vi "usbpt104+usbTC-arduino control PWM (RTD-TC PID).vi"() -> ()   [LabVIEW 2015]
uses:
  <vilib>/MakerHub/LINX/Public/Peripherals/Digital/Digital Write 1 Chan.vi
  <vilib>/MakerHub/LINX/Public/Peripherals/Digital/Digital Write N Chans.vi
  <vilib>/MakerHub/LINX/Private/Local IO/LinxDigitalWrite.vi
  <vilib>/MakerHub/LINX/Public/Utilities/Check Channel.vi
  Instance           1 16Saved   USBPT104 .vi
  <vilib>/MakerHub/LINX/Private/Utilties/Generate Error.vi
  <vilib>/MakerHub/LINX/LMH-LINX.lvlib
  UsbPT104.dll
  usbtc08.dll
panel:
  in  "RTD":bool
  out "Temperature":sgl
  out "RTD 4":dbl(slide) max=10000.0 scale=-200.0..800.0
  out "RTD 3":dbl(slide) max=10000.0 scale=-200.0..800.0
  out "RTD 2":dbl(slide) max=10000.0 scale=-200.0..800.0
  in  "PT104 Connection":bool=TRUE
  in  "IP Address":string
  out "Low Pulse Duration (ms)":dbl
  in  "Relay I/O Pin":u8
  in  "Update settings":bool
  in  "Stop":bool
  in  "PID":T1={"proportional gain (Kc)"=5.0, "integral time (Ti, min)"=0.0, "derivative time (Td, min)"=0.0}
  out "Data Saving...":bool caption="Saving Data"
  in  "Enable Save?":bool=TRUE caption="Enable"
  out "CH 8":sgl
  out "CH 7":sgl
  out "CH 6":sgl
  out "CH 5":sgl
  out "CH 4":sgl
  out "CH 3":sgl
  out "CH 2":sgl
  out "CH 1":sgl
  out "CH 0":sgl
  in  "Mains Frequency":i16(ring) items=["50 Hz", "60 Hz"]
  out "Handle":i16
  in  "?":bool
  in  "Units":enum16{"C°", "F°", "K°", "R°"}(ring)
  in  "Ch # 8":bool
  in  "Type # 8":i16(ring)=107 items=["B"=98, "E"=101, "J"=106, "K"=107, "N"=110, "R"=114, "S"=115, "T"=116, "Voltage"=120]
  in  "Ch # 7":bool
  in  "Type # 7":i16(ring)=107 items=["B"=98, "E"=101, "J"=106, "K"=107, "N"=110, "R"=114, "S"=115, "T"=116, "Voltage"=120]
  in  "Ch # 6":bool
  in  "Type # 6":i16(ring)=107 items=["B"=98, "E"=101, "J"=106, "K"=107, "N"=110, "R"=114, "S"=115, "T"=116, "Voltage"=120]
  in  "Ch # 5":bool
  in  "Type # 5":i16(ring)=107 items=["B"=98, "E"=101, "J"=106, "K"=107, "N"=110, "R"=114, "S"=115, "T"=116, "Voltage"=120]
  in  "Ch # 4":bool
  in  "Type # 4":i16(ring)=107 items=["B"=98, "E"=101, "J"=106, "K"=107, "N"=110, "R"=114, "S"=115, "T"=116, "Voltage"=120]
  in  "Ch # 3":bool
  in  "Type # 3":i16(ring)=107 items=["B"=98, "E"=101, "J"=106, "K"=107, "N"=110, "R"=114, "S"=115, "T"=116, "Voltage"=120]
  in  "Ch# 2":bool=TRUE
  in  "Type # 2":i16(ring)=107 items=["B"=98, "E"=101, "J"=106, "K"=107, "N"=110, "R"=114, "S"=115, "T"=116, "Voltage"=120]
  in  "Ch# 1":bool=TRUE
  in  "Type # 1":i16(ring)=107 items=["B"=98, "E"=101, "J"=106, "K"=107, "N"=110, "R"=114, "S"=115, "T"=116, "Voltage"=120]
  in  "Arduino Comms Port":refnum<visa-resource-name>
  out "Pulse Duration (ms)":dbl
  in  "Duty Cycle Period (ms)":u32=1000
  out "Duty Cycle (%)":dbl format="%.2f"
  out "PWM":dynamicdata(graph) caption="Square"
  in  "PID Temp Setpoint":u16=13
  out "?":dynamicdata(graph)
  in  "CH4 Measurement Type":i32(ring) items=["OFF", "PT100", "PT1000", "Resistance to 375 Ohms", "Resistance to 10 kOhms", "Differential to 115 mV", "Differential to 2500 mV", "Single-ended to 115 mV", "Single-ended to 2500 mV"]
  in  "CH4 Number of Wires":i16(ring)=4 items=["2"=2, "3"=3, "4"=4]
  in  "CH3 Measurement Type":i32(ring) items=["OFF", "PT100", "PT1000", "Resistance to 375 Ohms", "Resistance to 10 kOhms", "Differential to 115 mV", "Differential to 2500 mV", "Single-ended to 115 mV", "Single-ended to 2500 mV"]
  in  "CH3 Number of Wires":i16(ring)=4 items=["2"=2, "3"=3, "4"=4]
  in  "CH2 Measurement Type":i32(ring) items=["OFF", "PT100", "PT1000", "Resistance to 375 Ohms", "Resistance to 10 kOhms", "Differential to 115 mV", "Differential to 2500 mV", "Single-ended to 115 mV", "Single-ended to 2500 mV"]
  in  "CH2 Number of Wires":i16(ring)=4 items=["2"=2, "3"=3, "4"=4]
  in  "CH1 Number of Wires":i16(ring)=2 items=["2"=2, "3"=3, "4"=4]
  in  "CH1 Measurement Type":i32(ring)=1 items=["OFF", "PT100", "PT1000", "Resistance to 375 Ohms", "Resistance to 10 kOhms", "Differential to 115 mV", "Differential to 2500 mV", "Single-ended to 115 mV", "Single-ended to 2500 mV"]
  out "RTD 1":dbl(slide) max=10000.0 scale=-200.0..800.0
  # "RTD Channel 1 (PID Driven)"
  # "RTD Channel 2"
  # "RTD Channel 3"
  # "RTD Channel 4"
  # "TC"
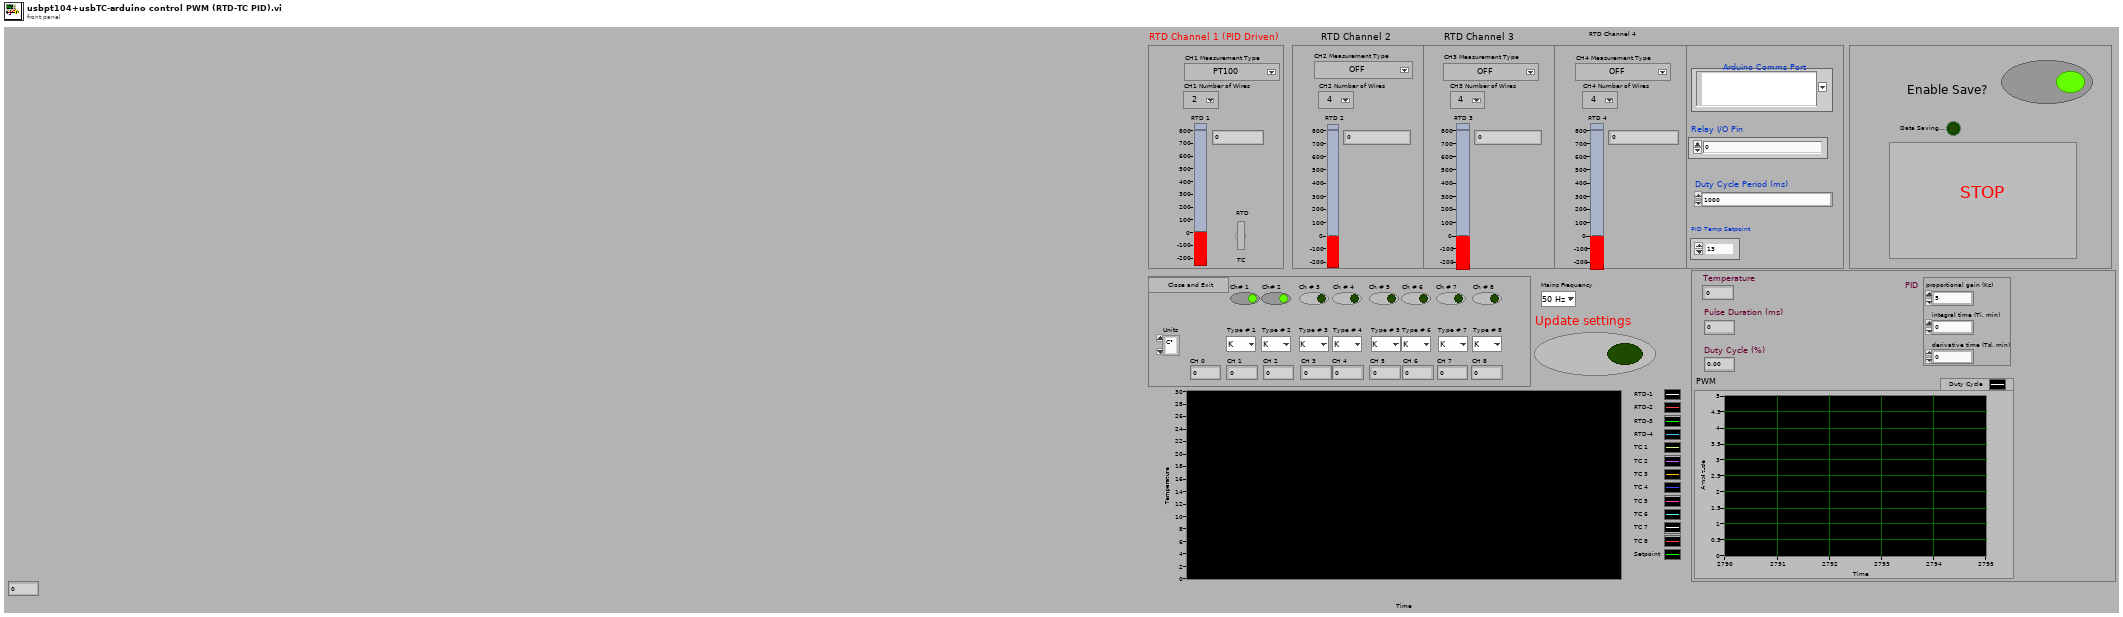
[diagram p1: front panel]
types:
  T1 = cluster{"proportional gain (Kc)":dbl, "integral time (Ti, min)":dbl, "derivative time (Td, min)":dbl}
  T2 = typedef "LMH-LINX.lvlib/LINX Ref.ctl" = cluster{"IO":T3, "Interface":T4, "LINX Device Config":T5}
  T3 = typedef "LMH-LINX.lvlib/Platform.ctl" = enum16{"Remote", "Local"}
  T4 = typedef "LMH-LINX.lvlib/Interface.ctl" = enum16{"Serial", "TCP"}
  T5 = typedef "LMH-LINX.lvlib/Device.lvlib/LINX Device Config.ctl" = cluster{"Interface":T4, "COM Port":refnum<visa-resource-name>, "TCP Configuration":T6, "Device Family":u8, "Device ID":u8, "Device Name":string, "TCP Ref":refnum<k5>, "Channels":T7}
  T6 = typedef "LMH-LINX.lvlib/Device.lvlib/TCP Config.ctl" = cluster{"IP Address":string, "Port":u16}
  T7 = typedef "LMH-LINX.lvlib/Channels.ctl" = cluster{"DI":u8[], "DO":u8[], "AI":u8[], "AO":u8[], "PWM":u8[], "QE":u8[], "UART":u8[], "I2C 2":u8[], "SPI":u8[], "CAN":u8[], "Servo":u8[], "AI Ref (V)":dbl, "AI Resolution (Bits)":u8, "AO Ref (V)":dbl, "AO Resolution (Bits)":u8}
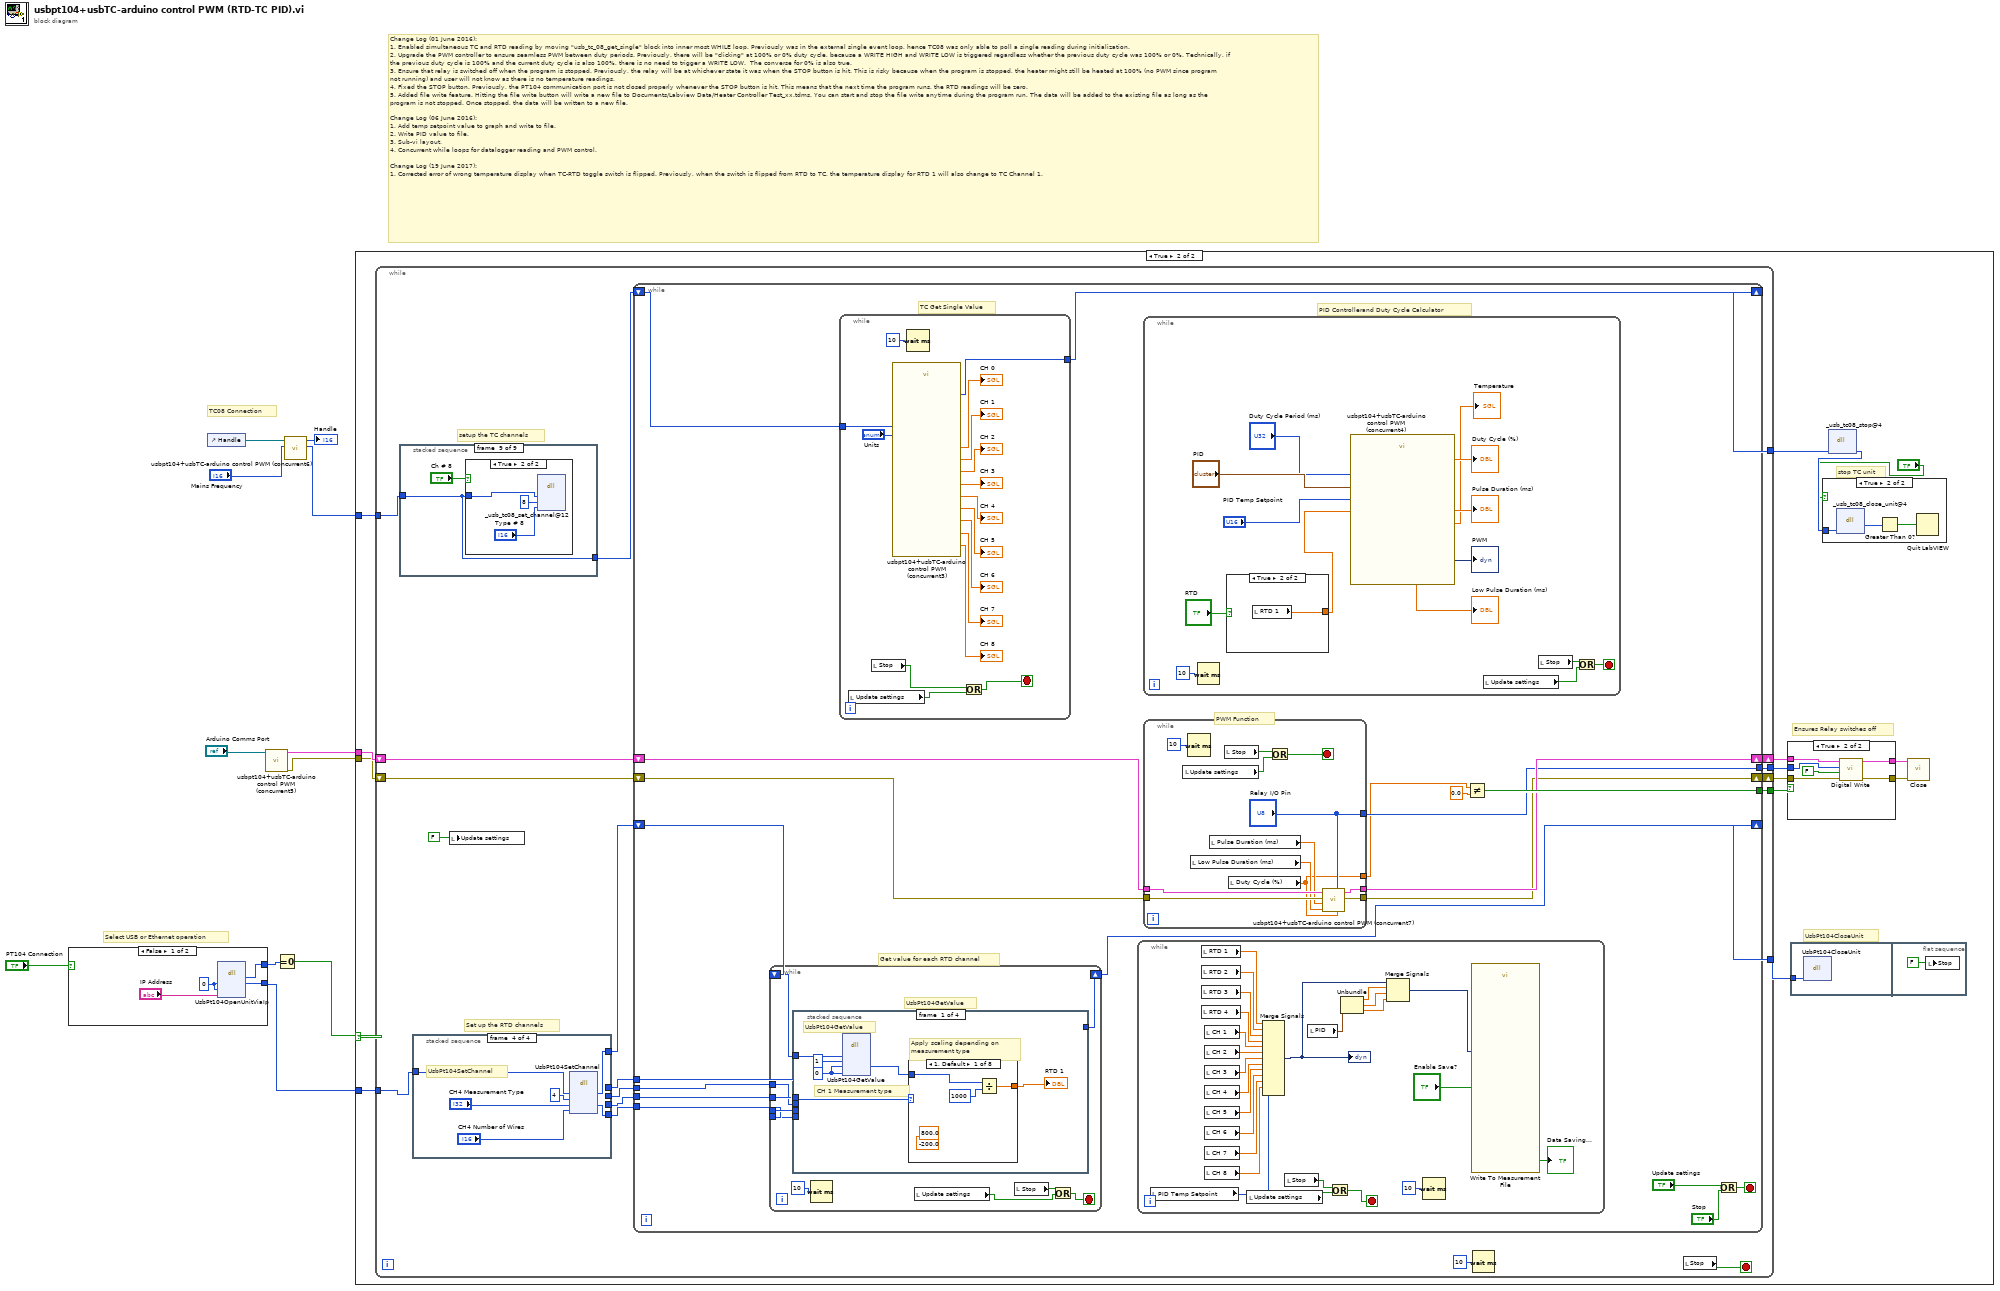
[diagram p0: block diagram]
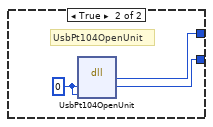
[diagram p2: hidden frame]
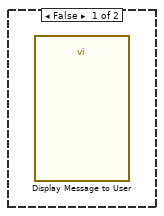
[diagram p3: hidden frame]
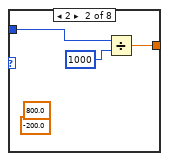
[diagram p4: hidden frame]
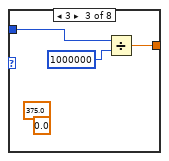
[diagram p5: hidden frame]
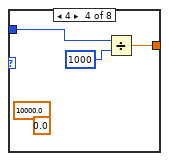
[diagram p6: hidden frame]
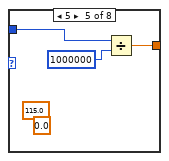
[diagram p7: hidden frame]
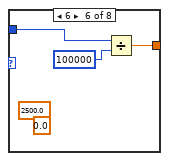
[diagram p8: hidden frame]
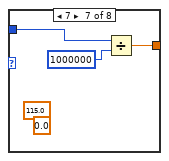
[diagram p9: hidden frame]
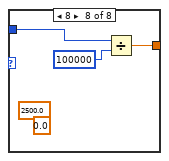
[diagram p10: hidden frame]
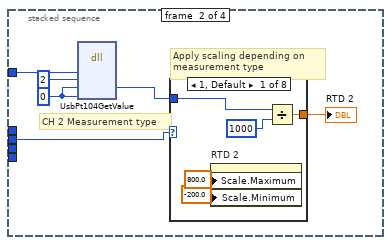
[diagram p11: hidden frame]
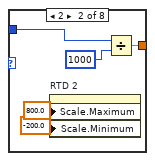
[diagram p12: hidden frame]
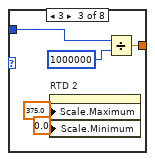
[diagram p13: hidden frame]
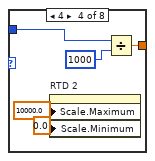
[diagram p14: hidden frame]
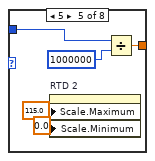
[diagram p15: hidden frame]
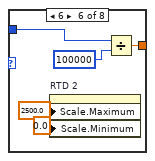
[diagram p16: hidden frame]
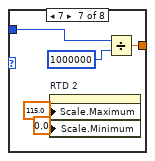
[diagram p17: hidden frame]
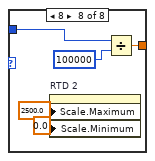
[diagram p18: hidden frame]
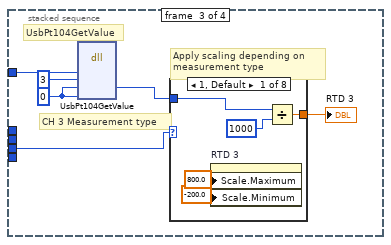
[diagram p19: hidden frame]
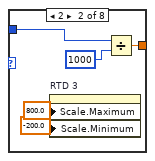
[diagram p20: hidden frame]
diagram:
  # "Select USB or Ethernet operation"
  # "TC08 Connection"
  # "Change Log (01 June 2016):\n1. Enabled simultaneous TC and RTD reading by moving \"usb_tc_08_get_single\" block into inner most WHILE loop. Previously was in the external single event loop, hence TC08 was only able to poll a single reading during initialization.\n2. Upgrade the PWM controller to ensure seamless PWM between duty periods. Previously, there will be \"clicking\" at 100% or 0% duty cycle, because a WRITE HIGH and WRITE LOW is triggered regardless whether the previous duty cycle was 100% or 0%. Technically, if the previous duty cycle is 100% and the current duty cycle is also 100%, there is no need to trigger a WRITE LOW.  The converse for 0% is also true. \n3. Ensure that relay is switched off when the program is stopped. Previously, the relay will be at whichever state it was when the STOP button is hit. This is risky because when the program is stopped, the heater might still be heated at 100% (no PWM since program not running) and user will not know as there is no temperature readings.\n4. Fixed the STOP button. Previously, the PT104 communication port is not closed properly whenever the STOP button is hit. This means that the next time the program runs, the RTD readings will be zero.\n5. Added file write feature. Hitting the file write button will write a new file to Documents/Labview Data/Heater Controller Test_xx.tdms. You can start and stop the file write anytime during the program run. The data will be added to the existing file as long as the program is not stopped. Once stopped, the data will be written to a new file. \n\nChange Log (06 June 2016):\n1. Add temp setpoint value to graph and write to file.\n2. Write PID value to file.\n3. Sub-vi layout.\n4. Concurrent while loops for datalogger reading and PWM control.\n\nChange Log (19 June 2017):\n1. Corrected error of wrong temperature display when TC-RTD toggle switch is flipped. Previously, when the switch is flipped from RTD to TC, the temperature display for RTD 1 will also change to TC Channel 1."
  n1 = case shown="False" "PT104 Connection" {
    tunnel: [w13 w18] -> w3
    tunnel: [w12 w17] -> w2
    frame False {
      w15 = i16 0 ("handle")
      n2 = dll-call lib="UsbPT104.dll" fn="UsbPt104OpenUnitViaIp"("handle"=w15, "serial"=w15, "IpAddress"="IP Address") -> ("Status"=w13:i32, "handle"=w12:i16)  [unwired: 5 in, 2 out]
    }
    frame True {
      w16 = i16 0 ("handle")
      # "UsbPt104OpenUnit"
      n3 = dll-call lib="UsbPT104.dll" fn="UsbPt104OpenUnit"("handle"=w16, "serial"=w16) -> ("Status"=w18:i32, "handle"=w17:i16)  [unwired: 4 in, 2 out]
    }
  }
  n4 = control-ref of="Handle"() -> (w9:refnum<vi>)
  n5 = call "usbpt104+usbTC-arduino control PWM (concurrent5).vi"("Arduino Comms Port"="Arduino Comms Port") -> ("error out"=w5:errorcluster, "LINX Resource"=w6:T2)  [unwired: 8 in]
  n6 = Equal To 0?(x=w3) -> (x = 0?=w1:bool)
  n7 = call "usbpt104+usbTC-arduino control PWM (concurrent6).vi"("Mains Frequency"="Mains Frequency", "Digital in"=w9) -> ("Handle 2"=w7:i16, "Handle"=→"Handle":i16)  [unwired: 8 in]
  n8 = case shown="True" w1 {
    tunnel: w7 -> [_ w27]
    tunnel: w2 -> [_ w19]
    tunnel: w6 -> [_ w24]
    tunnel: w5 -> [_ w22]
    frame False {
      n9 = call "Display Message to User"() -> ()  [unwired: 10 in, 2 out]
    }
    frame True {
      # "Ensures Relay switches off"
      # "UsbPt104CloseUnit"
      # "stop TC unit"
      n10 = while {
        tunnel: [w51] -> w28
        tunnel: w27 -> [w45]
        tunnel: [w43] -> w26
        tunnel: [w42] -> w25
        tunnel: [w37] -> w20
        tunnel: w19 -> [w36]
        shift-right: [w40] -> w23
        shift-left: w24 -> [w41]
        shift-right: [w38] -> w21
        shift-left: w22 -> [w39]
        stop <- w35 stop-if-true
        # "Set up the RTD channels"
        # "setup the TC channels"
        n11 = stacked-sequence {
          tunnel: [_ _ _ _ _ _ _ _ w399] -> w44
          tunnel: w45 -> [w340 w343 w351 w359 w367 w375 w383 w391 w399]
          frame #0 {
            n12 = dll-call lib="usbtc08.dll" fn="_usb_tc08_set_channel@12"("handle"=w340, "channel"=i16 0, "tc_type"=i8 0) -> ()  [unwired: 7 in, 2 out]
          }
          frame #1 {
            n13 = case shown="True" "Ch# 1" {
              tunnel: w343 -> [w346 w348]
              frame False {
                n14 = dll-call lib="usbtc08.dll" fn="_usb_tc08_set_channel@12"("handle"=w346, "channel"=i16 1, "tc_type"=32) -> ()  [unwired: 7 in, 2 out]
              }
              frame True {
                n15 = dll-call lib="usbtc08.dll" fn="_usb_tc08_set_channel@12"("handle"=w348, "channel"=i16 1, "tc_type"="Type # 1") -> ()  [unwired: 7 in, 2 out]
              }
            }
          }
          frame #2 {
            n16 = case shown="False" "Ch# 2" {
              tunnel: w351 -> [w353 w357]
              frame False {
                n17 = dll-call lib="usbtc08.dll" fn="_usb_tc08_set_channel@12"("handle"=w353, "channel"=i16 2, "tc_type"=32) -> ()  [unwired: 7 in, 2 out]
              }
              frame True {
                n18 = dll-call lib="usbtc08.dll" fn="_usb_tc08_set_channel@12"("handle"=w357, "channel"=i16 2, "tc_type"="Type # 2") -> ()  [unwired: 7 in, 2 out]
              }
            }
          }
          frame #3 {
            n19 = case shown="True" "Ch # 3" {
              tunnel: w359 -> [w361 w365]
              frame False {
                n20 = dll-call lib="usbtc08.dll" fn="_usb_tc08_set_channel@12"("handle"=w361, "channel"=i16 3, "tc_type"=32) -> ()  [unwired: 7 in, 2 out]
              }
              frame True {
                n21 = dll-call lib="usbtc08.dll" fn="_usb_tc08_set_channel@12"("handle"=w365, "channel"=i16 3, "tc_type"="Type # 3") -> ()  [unwired: 7 in, 2 out]
              }
            }
          }
          frame #4 {
            n22 = case shown="False" "Ch # 4" {
              tunnel: w367 -> [w369 w373]
              frame False {
                n23 = dll-call lib="usbtc08.dll" fn="_usb_tc08_set_channel@12"("handle"=w369, "channel"=i16 4, "tc_type"=32) -> ()  [unwired: 7 in, 2 out]
              }
              frame True {
                n24 = dll-call lib="usbtc08.dll" fn="_usb_tc08_set_channel@12"("handle"=w373, "channel"=i16 4, "tc_type"="Type # 4") -> ()  [unwired: 7 in, 2 out]
              }
            }
          }
          frame #5 {
            n25 = case shown="False" "Ch # 5" {
              tunnel: w375 -> [w377 w380]
              frame False {
                n26 = dll-call lib="usbtc08.dll" fn="_usb_tc08_set_channel@12"("handle"=w377, "channel"=i16 5, "tc_type"=32) -> ()  [unwired: 7 in, 2 out]
              }
              frame True {
                n27 = dll-call lib="usbtc08.dll" fn="_usb_tc08_set_channel@12"("handle"=w380, "channel"=i16 5, "tc_type"="Type # 5") -> ()  [unwired: 7 in, 2 out]
              }
            }
          }
          frame #6 {
            n28 = case shown="False" "Ch # 6" {
              tunnel: w383 -> [w385 w389]
              frame False {
                n29 = dll-call lib="usbtc08.dll" fn="_usb_tc08_set_channel@12"("handle"=w385, "channel"=i16 6, "tc_type"=32) -> ()  [unwired: 7 in, 2 out]
              }
              frame True {
                n30 = dll-call lib="usbtc08.dll" fn="_usb_tc08_set_channel@12"("handle"=w389, "channel"=i16 6, "tc_type"="Type # 6") -> ()  [unwired: 7 in, 2 out]
              }
            }
          }
          frame #7 {
            n31 = case shown="False" "Ch # 7" {
              tunnel: w391 -> [w393 w397]
              frame False {
                n32 = dll-call lib="usbtc08.dll" fn="_usb_tc08_set_channel@12"("handle"=w393, "channel"=i16 7, "tc_type"=32) -> ()  [unwired: 7 in, 2 out]
              }
              frame True {
                n33 = dll-call lib="usbtc08.dll" fn="_usb_tc08_set_channel@12"("handle"=w397, "channel"=i16 7, "tc_type"="Type # 7") -> ()  [unwired: 7 in, 2 out]
              }
            }
          }
          frame #8 {
            n34 = case shown="True" "Ch # 8" {
              tunnel: w399 -> [w401 w405]
              frame False {
                n35 = dll-call lib="usbtc08.dll" fn="_usb_tc08_set_channel@12"("handle"=w401, "channel"=i16 8, "tc_type"=32) -> ()  [unwired: 7 in, 2 out]
              }
              frame True {
                n36 = dll-call lib="usbtc08.dll" fn="_usb_tc08_set_channel@12"("handle"=w405, "channel"=i16 8, "tc_type"="Type # 8") -> ()  [unwired: 7 in, 2 out]
              }
            }
          }
        }
        n37 = stacked-sequence {
          tunnel: w36 -> [w323 w328 w333 w339]
          tunnel: [_ _ _ w335] -> w49
          tunnel: [w319 _ _ _] -> w50
          tunnel: [_ w324 _ _] -> w47
          tunnel: [_ _ w329 _] -> w46
          tunnel: [_ _ _ w334] -> w48
          frame #0 {
            # "UsbPt104SetChannel"
            n38 = dll-call lib="UsbPT104.dll" fn="UsbPt104SetChannel"("handle"=w323, "channel"=1, "type"="CH1 Measurement Type", "noOfWires"="CH1 Number of Wires") -> ("type"=w319:i32)  [unwired: 7 in, 2 out]
          }
          frame #1 {
            n39 = dll-call lib="UsbPT104.dll" fn="UsbPt104SetChannel"("handle"=w328, "channel"=2, "type"="CH2 Measurement Type", "noOfWires"="CH2 Number of Wires") -> ("type"=w324:i32)  [unwired: 7 in, 2 out]
          }
          frame #2 {
            # "UsbPt104SetChannel"
            n40 = dll-call lib="UsbPT104.dll" fn="UsbPt104SetChannel"("handle"=w333, "channel"=3, "type"="CH3 Measurement Type", "noOfWires"="CH3 Number of Wires") -> ("type"=w329:i32)  [unwired: 7 in, 2 out]
          }
          frame #3 {
            # "UsbPt104SetChannel"
            n41 = dll-call lib="UsbPT104.dll" fn="UsbPt104SetChannel"("handle"=w339, "channel"=4, "type"="CH4 Measurement Type", "noOfWires"="CH4 Number of Wires") -> ("handle"=w335:i16, "type"=w334:i32)  [unwired: 6 in, 2 out]
          }
        }
        n42 = local write "Update settings"(FALSE ("Update settings")) -> ()
        n43 = while {
          tunnel: [w69] -> w51
          tunnel: w50 -> [w59]
          tunnel: w48 -> [w55]
          tunnel: w47 -> [w57]
          tunnel: w46 -> [w56]
          tunnel: [w62] -> w37
          shift-right: [w52] -> w42
          shift-left: w49 -> [w58]
          shift-right: [w67] -> w43
          shift-left: w44 -> [w68]
          shift-right: [w65] -> w40
          shift-left: w41 -> [w66]
          shift-right: [w63] -> w38
          shift-left: w39 -> [w64]
          stop <- w60 stop-if-true
          # "PID Controllerand Duty Cycle Calculator"
          # "PWM Function"
          # "TC Get Single Value"
          # "Get value for each RTD channel"
          n44 = while {
            tunnel: w59 -> [w80]
            tunnel: w57 -> [w78]
            tunnel: w56 -> [w77]
            tunnel: w55 -> [w76]
            shift-right: [w75] -> w52
            shift-left: w58 -> [w79]
            stop <- w72 stop-if-true
            # "UsbPt104GetValue"
            n45 = stacked-sequence {
              tunnel: w79 -> [w86 w116 w162 w209]
              tunnel: [_ _ _ w206] -> w75
              tunnel: w80 -> [w82 _ _ _]
              tunnel: w78 -> [_ w111 _ _]
              tunnel: w77 -> [_ _ w157 _]
              tunnel: w76 -> [_ _ _ w203]
              frame #0 {
                w84 = 0 ("value")
                # "CH 1 Measurement type"
                # "Apply scaling depending on \nmeasurement type"
                # "UsbPt104GetValue"
                n46 = dll-call lib="UsbPT104.dll" fn="UsbPt104GetValue"("handle"=w86, "channel"=1, "value"=w84, "filtered"=w84) -> ("value"=w83:i32)  [unwired: 7 in, 2 out]
                n47 = case shown="1, Default" w82 {
                  tunnel: w83 -> [w88 w91 w94 w97 w100 w103 w106 w109]
                  tunnel: [w87 w90 w93 w96 w99 w102 w105 w108] -> w81
                  frame 1, Default {
                    (unwired) -200.0 ("Scale.Range:Minimum")
                    (unwired) 800.0 ("Data Range:Maximum")
                    n48 = Divide(x=w88, y=1000) -> (x/y=w87:dbl)
                  }
                  frame 2 {
                    (unwired) -200.0 ("Scale.Range:Minimum")
                    (unwired) 800.0 ("Data Range:Maximum")
                    n49 = Divide(x=w91, y=1000) -> (x/y=w90:dbl)
                  }
                  frame 3 {
                    (unwired) 0.0 ("Scale.Range:Minimum")
                    (unwired) 375.0 ("Data Range:Maximum")
                    n50 = Divide(x=w94, y=1000000) -> (x/y=w93:dbl)
                  }
                  frame 4 {
                    (unwired) 0.0 ("Scale.Range:Minimum")
                    (unwired) 10000.0 ("Data Range:Maximum")
                    n51 = Divide(x=w97, y=1000) -> (x/y=w96:dbl)
                  }
                  frame 5 {
                    (unwired) 0.0 ("Scale.Range:Minimum")
                    (unwired) 115.0 ("Data Range:Maximum")
                    n52 = Divide(x=w100, y=1000000) -> (x/y=w99:dbl)
                  }
                  frame 6 {
                    (unwired) 0.0 ("Scale.Range:Minimum")
                    (unwired) 2500.0 ("Data Range:Maximum")
                    n53 = Divide(x=w103, y=100000) -> (x/y=w102:dbl)
                  }
                  frame 7 {
                    (unwired) 0.0 ("Scale.Range:Minimum")
                    (unwired) 115.0 ("Data Range:Maximum")
                    n54 = Divide(x=w106, y=1000000) -> (x/y=w105:dbl)
                  }
                  frame 8 {
                    (unwired) 0.0 ("Scale.Range:Minimum")
                    (unwired) 2500.0 ("Data Range:Maximum")
                    n55 = Divide(x=w109, y=100000) -> (x/y=w108:dbl)
                  }
                }
                "RTD 1" <- w81
              }
              frame #1 {
                w114 = 0 ("value")
                # "CH 2 Measurement type"
                # "Apply scaling depending on \nmeasurement type"
                n56 = dll-call lib="UsbPT104.dll" fn="UsbPt104GetValue"("handle"=w116, "channel"=2, "value"=w114, "filtered"=w114) -> ("value"=w113:i32)  [unwired: 7 in, 2 out]
                n57 = case shown="1, Default" w111 {
                  tunnel: w113 -> [w120 w125 w130 w135 w140 w145 w150 w155]
                  tunnel: [w119 w124 w129 w134 w139 w144 w149 w154] -> w112
                  frame 1, Default {
                    n58 = property on="RTD 2" class="Slide (strict)"("Scale.Maximum"=800.0 ("Data Range:Maximum"), "Scale.Minimum"=-200.0 ("Scale.Range:Minimum")) -> ()  [unwired: 2 in, 2 out]
                    n59 = Divide(x=w120, y=1000) -> (x/y=w119:dbl)
                  }
                  frame 2 {
                    n60 = property on="RTD 2" class="Slide (strict)"("Scale.Maximum"=800.0 ("Data Range:Maximum"), "Scale.Minimum"=-200.0 ("Scale.Range:Minimum")) -> ()  [unwired: 2 in, 2 out]
                    n61 = Divide(x=w125, y=1000) -> (x/y=w124:dbl)
                  }
                  frame 3 {
                    n62 = property on="RTD 2" class="Slide (strict)"("Scale.Maximum"=375.0 ("Data Range:Maximum"), "Scale.Minimum"=0.0 ("Scale.Range:Minimum")) -> ()  [unwired: 2 in, 2 out]
                    n63 = Divide(x=w130, y=1000000) -> (x/y=w129:dbl)
                  }
                  frame 4 {
                    n64 = property on="RTD 2" class="Slide (strict)"("Scale.Maximum"=10000.0 ("Data Range:Maximum"), "Scale.Minimum"=0.0 ("Scale.Range:Minimum")) -> ()  [unwired: 2 in, 2 out]
                    n65 = Divide(x=w135, y=1000) -> (x/y=w134:dbl)
                  }
                  frame 5 {
                    n66 = property on="RTD 2" class="Slide (strict)"("Scale.Maximum"=115.0 ("Data Range:Maximum"), "Scale.Minimum"=0.0 ("Scale.Range:Minimum")) -> ()  [unwired: 2 in, 2 out]
                    n67 = Divide(x=w140, y=1000000) -> (x/y=w139:dbl)
                  }
                  frame 6 {
                    n68 = property on="RTD 2" class="Slide (strict)"("Scale.Maximum"=2500.0 ("Data Range:Maximum"), "Scale.Minimum"=0.0 ("Scale.Range:Minimum")) -> ()  [unwired: 2 in, 2 out]
                    n69 = Divide(x=w145, y=100000) -> (x/y=w144:dbl)
                  }
                  frame 7 {
                    n70 = property on="RTD 2" class="Slide (strict)"("Scale.Maximum"=115.0 ("Data Range:Maximum"), "Scale.Minimum"=0.0 ("Scale.Range:Minimum")) -> ()  [unwired: 2 in, 2 out]
                    n71 = Divide(x=w150, y=1000000) -> (x/y=w149:dbl)
                  }
                  frame 8 {
                    n72 = property on="RTD 2" class="Slide (strict)"("Scale.Maximum"=2500.0 ("Data Range:Maximum"), "Scale.Minimum"=0.0 ("Scale.Range:Minimum")) -> ()  [unwired: 2 in, 2 out]
                    n73 = Divide(x=w155, y=100000) -> (x/y=w154:dbl)
                  }
                }
                "RTD 2" <- w112
              }
              frame #2 {
                w160 = 0 ("value")
                # "CH 3 Measurement type"
                # "Apply scaling depending on \nmeasurement type"
                # "UsbPt104GetValue"
                n74 = dll-call lib="UsbPT104.dll" fn="UsbPt104GetValue"("handle"=w162, "channel"=3, "value"=w160, "filtered"=w160) -> ("value"=w159:i32)  [unwired: 7 in, 2 out]
                n75 = case shown="1, Default" w157 {
                  tunnel: w159 -> [w166 w171 w176 w181 w186 w191 w196 w201]
                  tunnel: [w165 w170 w175 w180 w185 w190 w195 w200] -> w158
                  frame 1, Default {
                    n76 = property on="RTD 3" class="Slide (strict)"("Scale.Maximum"=800.0 ("Data Range:Maximum"), "Scale.Minimum"=-200.0 ("Scale.Range:Minimum")) -> ()  [unwired: 2 in, 2 out]
                    n77 = Divide(x=w166, y=1000) -> (x/y=w165:dbl)
                  }
                  frame 2 {
                    n78 = property on="RTD 3" class="Slide (strict)"("Scale.Maximum"=800.0 ("Data Range:Maximum"), "Scale.Minimum"=-200.0 ("Scale.Range:Minimum")) -> ()  [unwired: 2 in, 2 out]
                    n79 = Divide(x=w171, y=1000) -> (x/y=w170:dbl)
                  }
                  frame 3 {
                    n80 = property on="RTD 3" class="Slide (strict)"("Scale.Maximum"=375.0 ("Data Range:Maximum"), "Scale.Minimum"=0.0 ("Scale.Range:Minimum")) -> ()  [unwired: 2 in, 2 out]
                    n81 = Divide(x=w176, y=1000000) -> (x/y=w175:dbl)
                  }
                  frame 4 {
                    n82 = property on="RTD 3" class="Slide (strict)"("Scale.Maximum"=10000.0 ("Data Range:Maximum"), "Scale.Minimum"=0.0 ("Scale.Range:Minimum")) -> ()  [unwired: 2 in, 2 out]
                    n83 = Divide(x=w181, y=1000) -> (x/y=w180:dbl)
                  }
                  frame 5 {
                    n84 = property on="RTD 3" class="Slide (strict)"("Scale.Maximum"=115.0 ("Data Range:Maximum"), "Scale.Minimum"=0.0 ("Scale.Range:Minimum")) -> ()  [unwired: 2 in, 2 out]
                    n85 = Divide(x=w186, y=1000000) -> (x/y=w185:dbl)
                  }
                  frame 6 {
                    n86 = property on="RTD 3" class="Slide (strict)"("Scale.Maximum"=2500.0 ("Data Range:Maximum"), "Scale.Minimum"=0.0 ("Scale.Range:Minimum")) -> ()  [unwired: 2 in, 2 out]
                    n87 = Divide(x=w191, y=100000) -> (x/y=w190:dbl)
                  }
                  frame 7 {
                    n88 = property on="RTD 3" class="Slide (strict)"("Scale.Maximum"=115.0 ("Data Range:Maximum"), "Scale.Minimum"=0.0 ("Scale.Range:Minimum")) -> ()  [unwired: 2 in, 2 out]
                    n89 = Divide(x=w196, y=1000000) -> (x/y=w195:dbl)
                  }
                  frame 8 {
                    n90 = property on="RTD 3" class="Slide (strict)"("Scale.Maximum"=2500.0 ("Data Range:Maximum"), "Scale.Minimum"=0.0 ("Scale.Range:Minimum")) -> ()  [unwired: 2 in, 2 out]
                    n91 = Divide(x=w201, y=100000) -> (x/y=w200:dbl)
                  }
                }
                "RTD 3" <- w158
              }
              frame #3 {
                w207 = 0 ("value")
                # "CH 4 Measurement type"
                # "Apply scaling depending on \nmeasurement type"
                # "UsbPt104GetValue"
                n92 = dll-call lib="UsbPT104.dll" fn="UsbPt104GetValue"("handle"=w209, "channel"=4, "value"=w207, "filtered"=w207) -> ("handle"=w206:i16, "value"=w205:i32)  [unwired: 6 in, 2 out]
                n93 = case shown="1, Default" w203 {
                  tunnel: w205 -> [w213 w218 w223 w228 w233 w238 w243 w248]
                  tunnel: [w212 w217 w222 w227 w232 w237 w242 w247] -> w204
                  frame 1, Default {
                    n94 = property on="RTD 4" class="Slide (strict)"("Scale.Maximum"=800.0 ("Data Range:Maximum"), "Scale.Minimum"=-200.0 ("Scale.Range:Minimum")) -> ()  [unwired: 2 in, 2 out]
                    n95 = Divide(x=w213, y=1000) -> (x/y=w212:dbl)
                  }
                  frame 2 {
                    n96 = property on="RTD 4" class="Slide (strict)"("Scale.Maximum"=800.0 ("Data Range:Maximum"), "Scale.Minimum"=-200.0 ("Scale.Range:Minimum")) -> ()  [unwired: 2 in, 2 out]
                    n97 = Divide(x=w218, y=1000) -> (x/y=w217:dbl)
                  }
                  frame 3 {
                    n98 = property on="RTD 4" class="Slide (strict)"("Scale.Maximum"=375.0 ("Data Range:Maximum"), "Scale.Minimum"=0.0 ("Scale.Range:Minimum")) -> ()  [unwired: 2 in, 2 out]
                    n99 = Divide(x=w223, y=1000000) -> (x/y=w222:dbl)
                  }
                  frame 4 {
                    n100 = property on="RTD 4" class="Slide (strict)"("Scale.Maximum"=10000.0 ("Data Range:Maximum"), "Scale.Minimum"=0.0 ("Scale.Range:Minimum")) -> ()  [unwired: 2 in, 2 out]
                    n101 = Divide(x=w228, y=1000) -> (x/y=w227:dbl)
                  }
                  frame 5 {
                    n102 = property on="RTD 4" class="Slide (strict)"("Scale.Maximum"=115.0 ("Data Range:Maximum"), "Scale.Minimum"=0.0 ("Scale.Range:Minimum")) -> ()  [unwired: 2 in, 2 out]
                    n103 = Divide(x=w233, y=1000000) -> (x/y=w232:dbl)
                  }
                  frame 6 {
                    n104 = property on="RTD 4" class="Slide (strict)"("Scale.Maximum"=2500.0 ("Data Range:Maximum"), "Scale.Minimum"=0.0 ("Scale.Range:Minimum")) -> ()  [unwired: 2 in, 2 out]
                    n105 = Divide(x=w238, y=100000) -> (x/y=w237:dbl)
                  }
                  frame 7 {
                    n106 = property on="RTD 4" class="Slide (strict)"("Scale.Maximum"=115.0 ("Data Range:Maximum"), "Scale.Minimum"=0.0 ("Scale.Range:Minimum")) -> ()  [unwired: 2 in, 2 out]
                    n107 = Divide(x=w243, y=1000000) -> (x/y=w242:dbl)
                  }
                  frame 8 {
                    n108 = property on="RTD 4" class="Slide (strict)"("Scale.Maximum"=2500.0 ("Data Range:Maximum"), "Scale.Minimum"=0.0 ("Scale.Range:Minimum")) -> ()  [unwired: 2 in, 2 out]
                    n109 = Divide(x=w248, y=100000) -> (x/y=w247:dbl)
                  }
                }
                "RTD 4" <- w204
              }
            }
            n110 = Wait (ms)(milliseconds to wait=u32 10) -> ()  [unwired: 1 out]
            n111 = local read "Update settings"() -> (w71:bool)
            n112 = local read "Stop"() -> (w73:bool)
            n113 = Or(x=w73, y=w71) -> (x .or. y?=w72:bool)
          }
          n114 = while {
            tunnel: w68 -> [w281]
            tunnel: [w280] -> w67
            stop <- w276 stop-if-true
            n115 = local read "Update settings"() -> (w275:bool)
            n116 = local read "Stop"() -> (w277:bool)
            n117 = call "usbpt104+usbTC-arduino control PWM (concurrent3).vi"("handle"=w281, "Units"="Units") -> ("CH 3"=→"CH 3":sgl, "CH 2"=→"CH 2":sgl, "CH 0"=→"CH 0":sgl, "CH 1"=→"CH 1":sgl, "handle 2"=w280:i16, "CH 4"=→"CH 4":sgl, "CH 8"=→"CH 8":sgl, "CH 5"=→"CH 5":sgl, "CH 6"=→"CH 6":sgl, "CH 7"=→"CH 7":sgl)
            n118 = Wait (ms)(milliseconds to wait=u32 10) -> ()  [unwired: 1 out]
            n119 = Or(x=w277, y=w275) -> (x .or. y?=w276:bool)
          }
          n120 = while {
            stop <- w259 stop-if-true
            n121 = local read "PID Temp Setpoint"() -> (w262:u16)
            n122 = local read "RTD 1"() -> (w274:dbl)
            n123 = local read "RTD 2"() -> (w273:dbl)
            n124 = local read "RTD 3"() -> (w272:dbl)
            n125 = local read "RTD 4"() -> (w271:dbl)
            n126 = local read "CH 1"() -> (w270:sgl)
            n127 = local read "CH 2"() -> (w269:sgl)
            n128 = local read "CH 3"() -> (w268:sgl)
            n129 = local read "CH 4"() -> (w267:sgl)
            n130 = local read "CH 5"() -> (w266:sgl)
            n131 = local read "CH 6"() -> (w265:sgl)
            n132 = local read "CH 7"() -> (w264:sgl)
            n133 = local read "CH 8"() -> (w263:sgl)
            n134 = local read "Update settings"() -> (w258:bool)
            n135 = Merge Signals(w274, w273, w272, w271, w270, w269, w268, w267, w266, w265, w264, w263, w262) -> (w255:dynamicdata)
            "?" <- w255
            n136 = local read "Stop"() -> (w260:bool)
            n137 = local read "PID"() -> (w254:T1)
            n138 = Or(x=w260, y=w258) -> (x .or. y?=w259:bool)
            n139 = Unbundle(w254) -> ("proportional gain (Kc)"=w253:dbl, "integral time (Ti, min)"=w252:dbl, "derivative time (Td, min)"=w251:dbl)
            n140 = Merge Signals(w255, w253, w252, w251) -> (w250:dynamicdata)
            n141 = Wait (ms)(milliseconds to wait=u32 10) -> ()  [unwired: 1 out]
            n142 = call "Write To Measurement File"("Signals"=w250, "Enable"="Enable Save?") -> ("Saving Data"=→"Data Saving...":bool)  [unwired: 15 in, 2 out]
          }
          n143 = while {
            stop <- w295 stop-if-true
            n144 = Wait (ms)(milliseconds to wait=u32 10) -> ()  [unwired: 1 out]
            n145 = case shown="True" "RTD" {
              tunnel: [w305 w306] -> w292
              frame False {
                n146 = local read "CH 1"() -> (w305:sgl)
              }
              frame True {
                n147 = local read "RTD 1"() -> (w306:dbl)
              }
            }
            n148 = call "usbpt104+usbTC-arduino control PWM (concurrent4).vi"("RTD 1 Temp Input"=w292, "PID"="PID", "PID Temp Setpoint"="PID Temp Setpoint", "Duty Cycle Period (ms)"="Duty Cycle Period (ms)") -> ("Low Pulse Duration (ms)"=→"Low Pulse Duration (ms)":dbl, "High Pulse Duration (ms)"=→"Pulse Duration (ms)":dbl, "Duty Cycle (%)"=→"Duty Cycle (%)":dbl, "PWM"=→"PWM":dynamicdata, "CH1 Value"=→"Temperature":dbl)  [unwired: 3 in]
            n149 = local read "Update settings"() -> (w294:bool)
            n150 = local read "Stop"() -> (w296:bool)
            n151 = Or(x=w296, y=w294) -> (x .or. y?=w295:bool)
          }
          n152 = while {
            tunnel: w66 -> [w318]
            tunnel: [w317] -> w65
            tunnel: w64 -> [w316]
            tunnel: [w315] -> w63
            tunnel: ["Relay I/O Pin"] -> w62
            tunnel: [w311] -> w54
            stop <- w309 stop-if-true
            n153 = local read "Update settings"() -> (w307:bool)
            n154 = Wait (ms)(milliseconds to wait=u32 10) -> ()  [unwired: 1 out]
            n155 = local read "Low Pulse Duration (ms)"() -> (w313:dbl)
            n156 = local read "Pulse Duration (ms)"() -> (w312:dbl)
            n157 = local read "Stop"() -> (w308:bool)
            n158 = local read "Duty Cycle (%)"() -> (w311:dbl)
            n159 = Or(x=w308, y=w307) -> (x .or. y?=w309:bool)
            n160 = call "usbpt104+usbTC-arduino control PWM (concurrent7).vi"("LINX Resource"=w318, "error in"=w316, "High Pulse Duration (ms)"=w312, "Low Pulse Duration"=w313, "Relay I/O Pin"="Relay I/O Pin", "Duty Cycle (%)"=w311) -> ("LINX Resource Out"=w317:T2, "Error Out"=w315:errorcluster)  [unwired: 2 in]
          }
          n161 = Not Equal?(x=w54, y=0.0) -> (x != y?=w69:bool)
          n162 = Or(x="Update settings", y="Stop") -> (x .or. y?=w60:bool)
        }
        n163 = Wait (ms)(milliseconds to wait=u32 10) -> ()  [unwired: 1 out]
        n164 = local read "Stop"() -> (w35:bool)
      }
      n165 = case shown="True" w28 {
        tunnel: w20 -> [_ w411]
        tunnel: w23 -> [w410 w416]
        tunnel: w21 -> [w409 w415]
        tunnel: [w410 w413] -> w30
        tunnel: [w409 w412] -> w29
        frame False {
        }
        frame True {
          n166 = call-poly <vilib>:"Digital Write.vi"("Error In"=w415, "Output Value"=FALSE, "DO Channel"=w411, "LINX Resource"=w416) -> ("Error Out"=w412:errorcluster, "LINX Resource"=w413:T2)  [unwired: 6 in]
        }
      }
      n167 = flat-sequence {
        tunnel: w25 -> [w407]
        frame #0 {
          n168 = dll-call lib="UsbPT104.dll" fn="UsbPt104CloseUnit"("handle"=w407) -> ()  [unwired: 5 in, 2 out]
        }
        frame #1 {
          n169 = local write "Stop"(FALSE ("Stop")) -> ()
        }
      }
      n170 = dll-call lib="usbtc08.dll" fn="_usb_tc08_stop@4" ("Close unit")("handle"=w26) -> ("handle"=w32:i16)  [unwired: 4 in, 2 out]
      n171 = case shown="True" "?" {
        tunnel: w32 -> [_ w419]
        frame False {
        }
        frame True {
          n172 = dll-call lib="usbtc08.dll" fn="_usb_tc08_close_unit@4" ("Close unit")("handle"=w419) -> (w418:i16)  [unwired: 4 in, 2 out]
          n173 = Greater Than 0?(x=w418) -> (x > 0?=w417:bool)
          n174 = Quit LabVIEW(quit? (T)=w417) -> ()
        }
      }
      n175 = call <vilib>:"Close.vi"("Error In"=w29, "LINX Resource"=w30) -> ()  [unwired: 9 in, 1 out]
    }
  }
